vi "Read.vi"(8 "error in (no error)":errorcluster, 11 "CVT_DBL in":refnum<class "CVT_DBL.lvclass">) -> (0 "error out":errorcluster, 2 "value":dbl, 3 "CVT_DBL out":refnum<class "CVT_DBL.lvclass">)   [LabVIEW 2024, in "Current Value Table.lvlib" / "CVT_DBL.lvclass"]
uses:
  CVT_DBL.lvclass
  CVT_DBL.lvclass/CVT_DBL.ctl
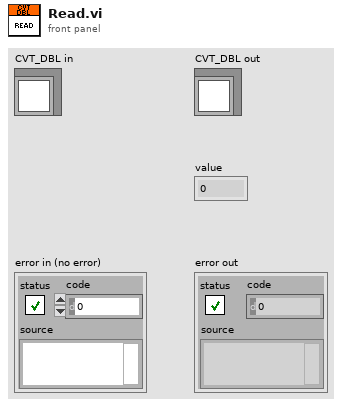
[diagram p1: front panel]
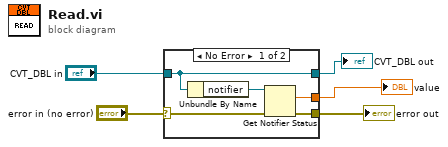
[diagram p0: block diagram]
diagram:
  n1 = case shown="No Error" "error in (no error)" {
    selector: "error in (no error)" -> [w7 w12]
    tunnel: [w6 w12] -> w4
    tunnel: [w10 w11] -> w2
    tunnel: "CVT_DBL in" -> [w10 w11]
    tunnel: [w8 _] -> w1
    frame No Error {
      n2 = Unbundle By Name(w10) -> ("notifier"=w9:refnum<notifier>)
      n3 = Get Notifier Status(notifier=w9, error in (no error)=w7) -> (current notification=w8:dbl, error out=w6:errorcluster)  [unwired: 3 out]
    }
    frame Error {
    }
  }
  "error out" <- w4
  "CVT_DBL out" <- w2
  "value" <- w1
